vi "Read name.vi"(9 "Node in":refnum<class "Node.lvclass">) -> (3 "Node out":refnum<class "Node.lvclass">, 4 "name":string)   [LabVIEW 2014, in "Raspberry Pi Compatible Compiler for LabVIEW.lvlib" / "Node.lvclass"]
uses:
  Node.lvclass
  Node.lvclass/Node.ctl
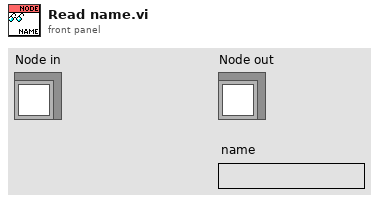
[diagram p1: front panel]
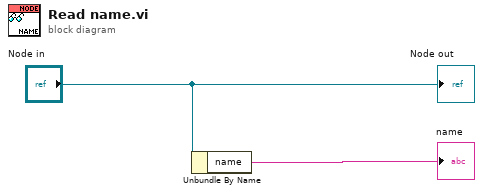
[diagram p0: block diagram]
diagram:
  n1 = Unbundle By Name("Node in") -> ("name"=→"name":string)
  "Node out" <- "Node in"
